vi "Pre Launch Init.vi"(11 "ChildActor in":refnum<class "ChildActor.lvclass"> caption="操作者输入") -> (0 "error out":errorcluster caption="错误输出", 3 "ChildActor out":refnum<class "ChildActor.lvclass"> caption="操作者输出")   [LabVIEW 2014, in "UnitTest.lvlib" / "ChildActor.lvclass"]
doc: "(<B>Filename</B>: Actor Framework.lvlib:Actor.lvclass:Pre Launch Init.vi)\n\nDefines behavior that occurs after the Launch Nested Actor method is invoked but before the actor's Actor Core method begins running.\n\nBy default, this method does nothing. A descendant class may override it to define behavior."
uses:
  ChildActor.lvclass
  <vilib>/ActorFramework/Actor/Actor.lvclass
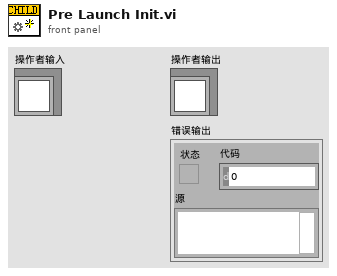
[diagram p1: front panel]
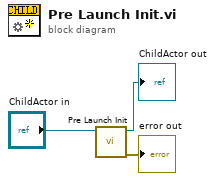
[diagram p0: block diagram]
diagram:
  n1 = call-parent "Pre Launch Init.vi"("Actor in"="ChildActor in") -> ("error out"=→"error out":errorcluster, "Actor out"=→"ChildActor out":refnum<class "ChildActor.lvclass">)  [unwired: 9 in]
